vi "test-worker mode.vi"(8 "error in (no error)":errorcluster, 11 "TestCase in":refnum<class "testcase-CSMAttributes.lvclass">) -> (0 "error out":errorcluster, 3 "TestCase out":refnum<class "testcase-CSMAttributes.lvclass">)   [LabVIEW 2017, in "testcase-CSMAttributes.lvclass"]
uses:
  testcase-CSMAttributes.lvclass
  6faf3dd6-bbe3-43e6-ac0e-6a595a4bbb73.vi
  eea55257-98dc-4069-a2fc-7f3abec53d34.vi
  654a1434-e049-45b7-bbe1-b3daff27deed.vi
  232dea5e-886f-41b8-bb39-dacd9565842e.vi
  d39486ea-fbfe-4c2b-b0ae-85d31efdfc25.vi
  4fbfc3b2-4ab6-4b17-950e-362f3a1418f9.vi
  eb53d3db-f5cc-4d50-900d-3a282fe3921b.vi
  d3eb8ef0-7d19-473b-ace2-fe9805f10b86.vi
  src/user.lib/_NEVSTOP/Communicable State Machine(CSM)/AdvanceAPI/CSM - Set Module Attribute.vi
  src/user.lib/_NEVSTOP/Communicable State Machine(CSM)/AdvanceAPI/CSM - Get Module Attribute.vi
  src/user.lib/_NEVSTOP/Communicable State Machine(CSM)/Communicable State Machine.lvlib
  <vilib>/addons/_JKI Toolkits/VI Tester/TestCase.llb/TestCase.lvclass
  C:/Program Files (x86)/National Instruments/LabVIEW 2017/vi.lib/addons/_JKI Toolkits/VI Tester/TestCase.llb/TestCase.lvclass
panel:
  out "Error out":errorcluster
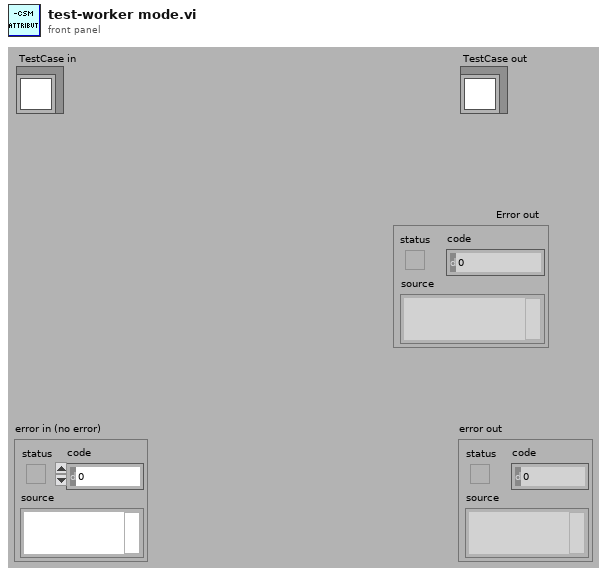
[diagram p1: front panel]
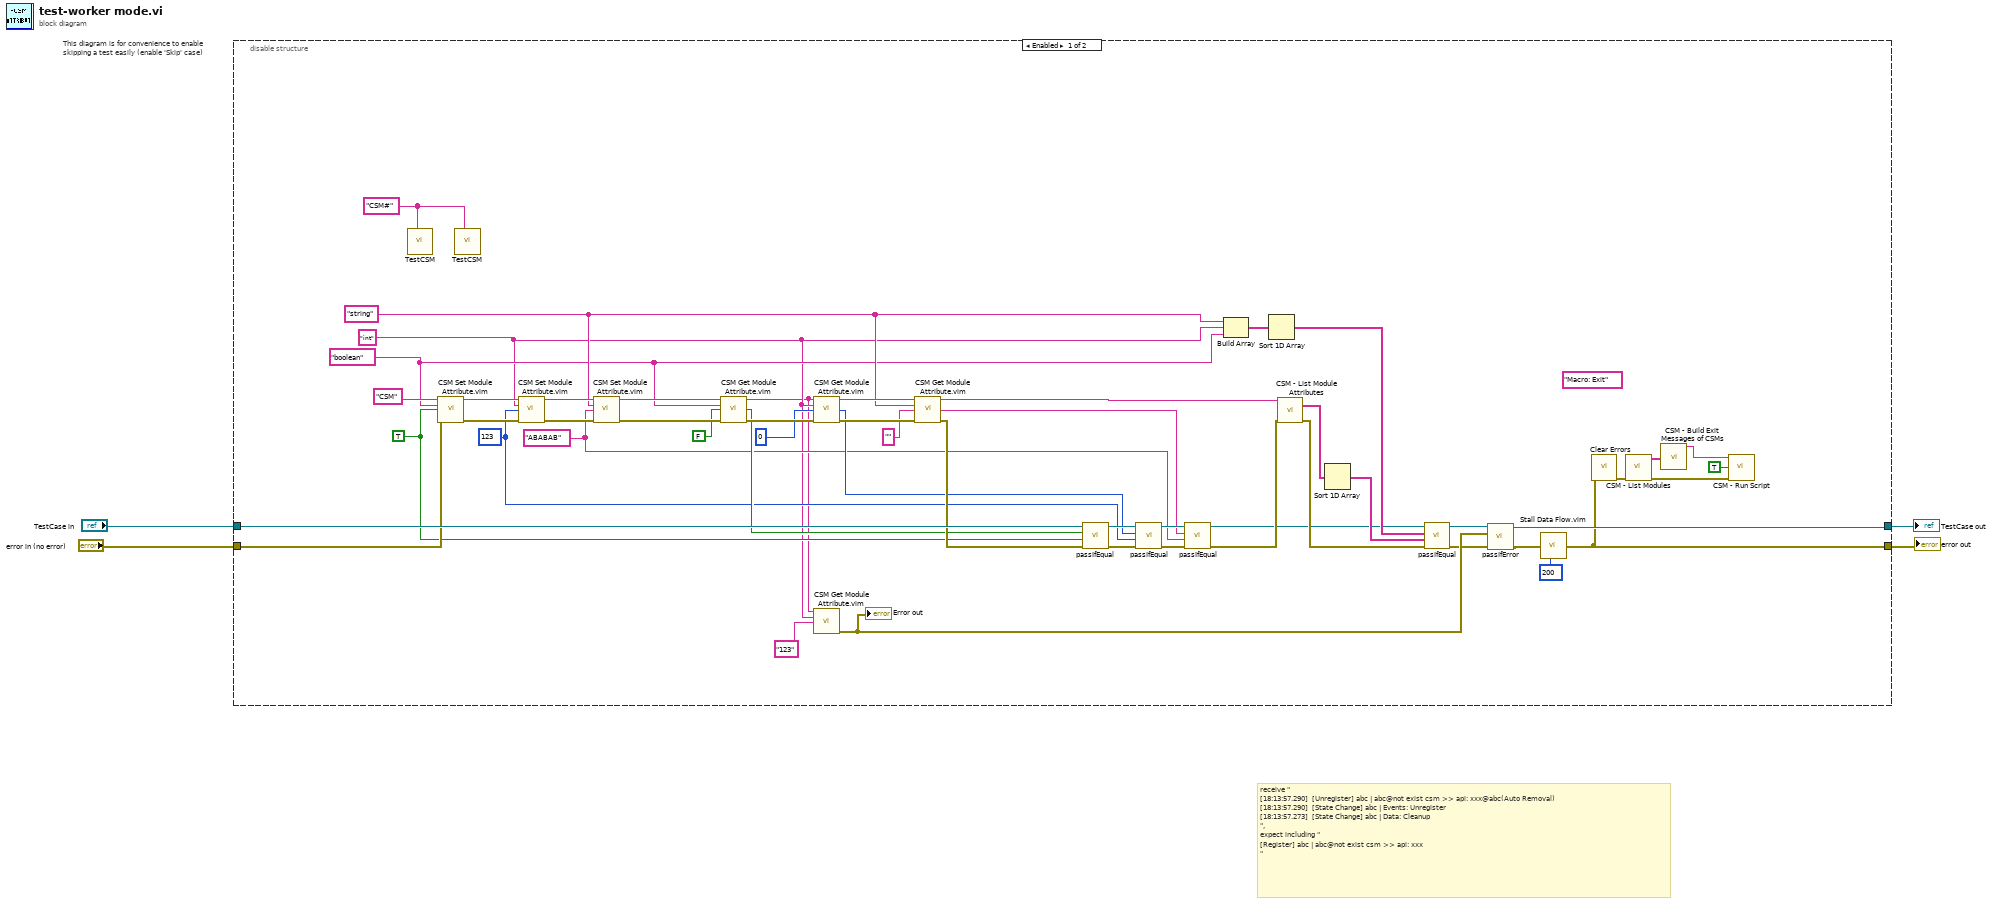
[diagram p0: block diagram]
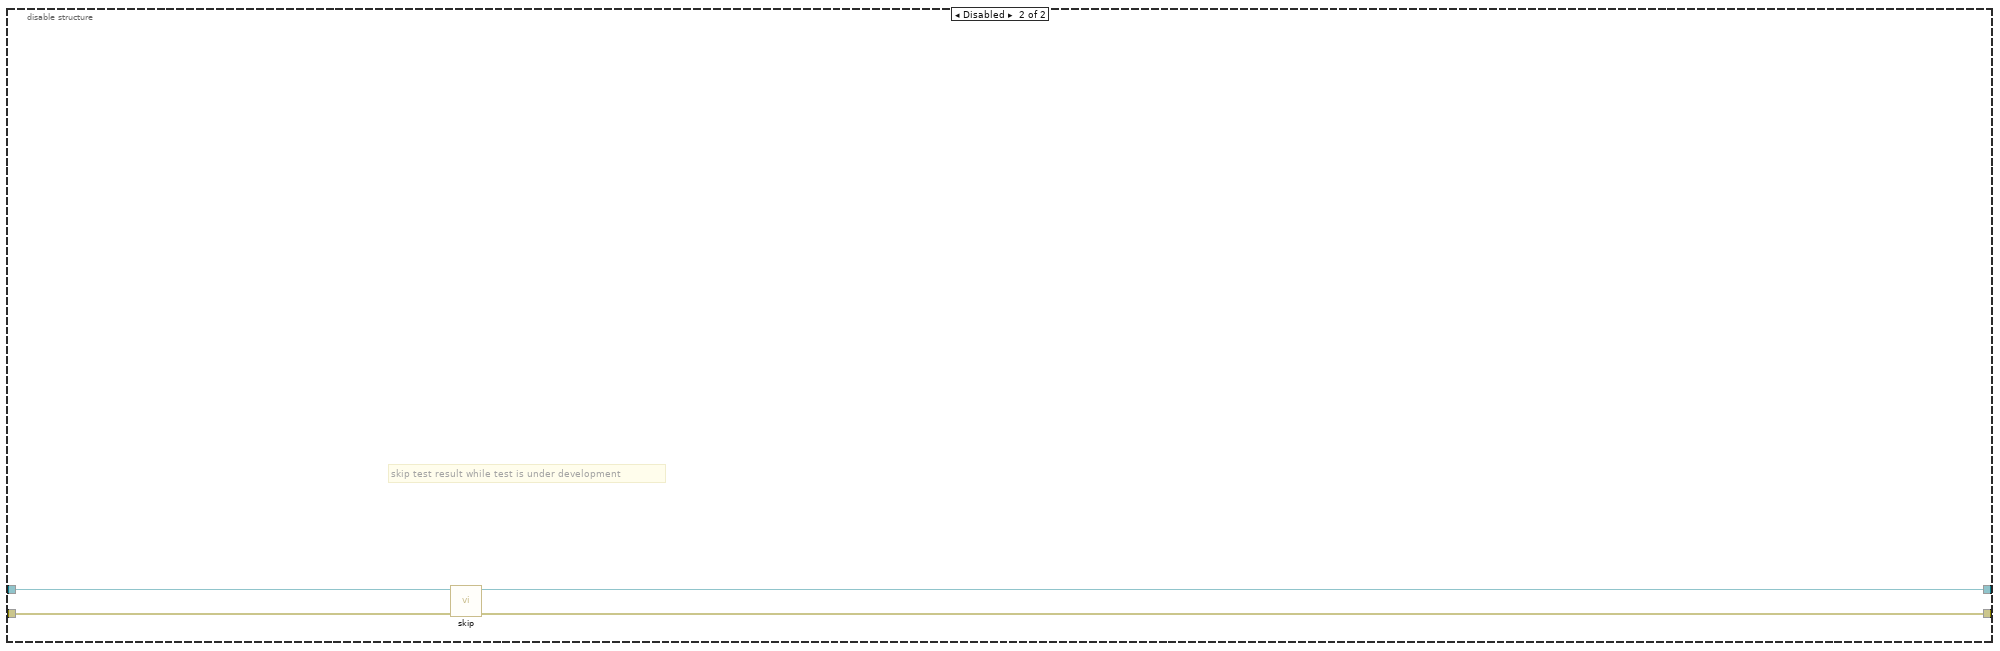
[diagram p2: hidden frame]
diagram:
  # "receive \"\n[18:13:57.290]  [Unregister] abc | abc@not exist csm >> api: xxx@abc(Auto Removal)\n[18:13:57.290]  [State Change] abc | Events: Unregister\n[18:13:57.273]  [State Change] abc | Data: Cleanup\n\", \nexpect including \"\n[Register] abc | abc@not exist csm >> api: xxx\n\""
  n1 = disable-structure "This diagram is for convenience to enable skipping a test easily (enable 'Skip' case)" shown="Enabled" {
    disable-tunnel: "TestCase in" -> [w56 w60]
    disable-tunnel: [w12 w58] -> w1
    disable-tunnel: [w6 w59] -> w3
    disable-tunnel: "error in (no error)" -> [w55 w57]
    frame Enabled {
      (unwired) "Macro: Exit" ("State")
      w31 = "ABABAB" ("Attribute")
      w27 = "string" ("Attribute")
      w35 = 123
      w18 = "int" ("Attribute")
      w40 = TRUE
      w26 = "boolean" ("Attribute")
      w11 = "CSM#" ("Name(\"\" to use uuid)")
      n2 = call "TestCSM.vi"("Name(\"\" to use uuid)"=w11) -> ()  [unwired: 11 in]
      n3 = call "CSM Set Module Attribute.vim"("CSM Name"="CSM" ("Name(\"\" to use uuid)"), "Attribute"=w26, "value"=w40, "Error in"=w55) -> ("CSM Name(dup)"=w51:string, "Error out"=w53:errorcluster)  [unwired: 8 in, 2 out]
      n4 = call "TestCSM.vi"("Name(\"\" to use uuid)"=w11) -> ()  [unwired: 11 in]
      n5 = call "CSM Set Module Attribute.vim"("CSM Name"=w51, "Attribute"=w18, "value"=w35, "Error in"=w53) -> ("CSM Name(dup)"=w50:string, "Error out"=w52:errorcluster)  [unwired: 8 in, 2 out]
      n6 = call "CSM Set Module Attribute.vim"("CSM Name"=w50, "Attribute"=w27, "value"=w31, "Error in"=w52) -> ("CSM Name(dup)"=w48:string, "Error out"=w49:errorcluster)  [unwired: 8 in, 2 out]
      n7 = call "CSM Get Module Attribute.vim"("CSM Name"=w48, "Attribute"=w26, "default value (empty variant)"=FALSE, "Error in"=w49) -> ("CSM Name(dup)"=w17:string, "value"=w39:bool, "Error out"=w47:errorcluster)  [unwired: 7 in, 2 out]
      n8 = call "CSM Get Module Attribute.vim"("CSM Name"=w17, "Attribute"=w18, "default value (empty variant)"=0, "Error in"=w47) -> ("CSM Name(dup)"=w46:string, "value"=w36:i32, "Error out"=w45:errorcluster)  [unwired: 7 in, 2 out]
      n9 = call "CSM Get Module Attribute.vim"("CSM Name"=w17, "Attribute"=w18, "default value (empty variant)"="123") -> ("Error out"=w15:errorcluster)  [unwired: 8 in, 4 out]
      "Error out" <- w15
      n10 = call "CSM Get Module Attribute.vim"("CSM Name"=w46, "Attribute"=w27, "default value (empty variant)"="" ("Attribute"), "Error in"=w45) -> ("CSM Name(dup)"=w30:string, "value"=w32:string, "Error out"=w41:errorcluster)  [unwired: 7 in, 2 out]
      n11 = call-dynamic "passIfEqual.vi"("error in (no error)"=w41, "y"=w40, "x"=w39, "TestCase in"=w56) -> ("error out"=w37:errorcluster, "TestCase out"=w38:refnum<class "testcase-CSMAttributes.lvclass">)  [unwired: 6 in]
      n12 = call-dynamic "passIfEqual.vi"("error in (no error)"=w37, "y"=w35, "x"=w36, "TestCase in"=w38) -> ("error out"=w33:errorcluster, "TestCase out"=w34:refnum<class "testcase-CSMAttributes.lvclass">)  [unwired: 6 in]
      n13 = call-dynamic "passIfEqual.vi"("error in (no error)"=w33, "y"=w31, "x"=w32, "TestCase in"=w34) -> ("error out"=w29:errorcluster, "TestCase out"=w21:refnum<class "testcase-CSMAttributes.lvclass">)  [unwired: 6 in]
      n14 = Build Array(w27, w18, w26) -> (w25:string[])
      n15 = Sort 1D Array(array=w25) -> (sorted array=w22:string[])
      n16 = call "CSM - List Module Attributes.vi"("CSM Name"=w30, "Error in"=w29) -> ("Attributes"=w24:string[], "Error out"=w28:errorcluster)  [unwired: 9 in, 3 out]
      n17 = Sort 1D Array(array=w24) -> (sorted array=w23:string[])
      n18 = call-dynamic "passIfEqual.vi"("error in (no error)"=w28, "y"=w23, "x"=w22, "TestCase in"=w21) -> ("error out"=w14:errorcluster, "TestCase out"=w16:refnum<class "testcase-CSMAttributes.lvclass">)  [unwired: 6 in]
      n19 = call-dynamic "passIfError.vi"("error in (no error)"=w14, "error"=w15, "TestCase in"=w16) -> ("error out"=w13:errorcluster, "TestCase out"=w12:refnum<class "testcase-CSMAttributes.lvclass">)  [unwired: 7 in]
      n20 = call "Stall Data Flow.vim"("value in"=w13, "milliseconds to wait"=u32 200) -> ("value out"=w6:errorcluster)  [unwired: 1 out]
      n21 = call <vilib>:"Clear Errors.vi"("error in (no error)"=w6) -> ("error out"=w20:errorcluster)  [unwired: 5 in, 1 out]
      n22 = call "CSM - List Modules.vi"("Error in"=w20) -> ("Error out"=w10:errorcluster, "Module Names"=w9:string[])  [unwired: 9 in]
      n23 = call "CSM - Build Exit Messages of CSMs.vi"("CSMs"=w9) -> ("States"=w7:string)  [unwired: 14 in]
      n24 = call "CSM - Run Script.vi"("CSM Scripts"=w7, "Continue If Error?(F)"=TRUE, "error in (no error)"=w10) -> ()  [unwired: 10 in, 3 out]
    }
    frame Disabled {
      # "skip test result while test is under development"
      n25 = call <vilib>:"skip.vi"("error in (no error)"=w57, "TestCase in"=w60) -> ("error out"=w59:errorcluster, "TestCase out"=w58:refnum<class "testcase-CSMAttributes.lvclass">)  [unwired: 8 in]
    }
  }
  "error out" <- w3
  "TestCase out" <- w1
